vi "Panel.vi"(11 "PlatformArrayPanel in":refnum<class "PlatformArrayPanel.lvclass">) -> ()   [LabVIEW 2020, in "PicoG-App.lvlib" / "PlatformArrayPanel.lvclass"]
uses:
  PlatformArrayPanel.lvclass
  C:/Program Files (x86)/National Instruments/LabVIEW 2020/vi.lib/IlluminatedG/IG OOPanel/OOPanel/Panel/Panel.lvclass
  <vilib>/IlluminatedG/IG OOPanel/OOPanel/Panel/Basic UI State.ctl
  PlatformArrayPanel.lvclass/PlatformArrayPanel.ctl
  Builds/picoG/ppl/PicoG-Core.lvlibp/PicoG-Processor/PicoG-Core/DeployPlatform/DeployPlatform.lvclass
  <vilib>/IlluminatedG/IG OOPanel/OOPanel/Panel/Panel.lvclass
  <vilib>/IlluminatedG/IG OOPanel/OOPanel/OOPanel.lvlib
  C:/Program Files (x86)/National Instruments/LabVIEW 2020/vi.lib/IlluminatedG/IG OOPanel/OOPanel/ArrayPanel/ArrayPanel.lvclass
  C:/dev/Vireo/PicoG/PicoG-App/PlatformArrayPanel/PlatformArrayPanel.lvclass
panel:
  out "Name":string
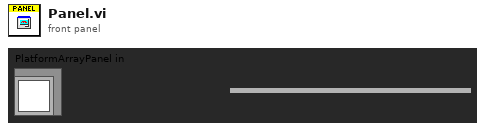
[diagram p1: front panel]
types:
  T1 = typedef "OOPanel.lvlib/Panel.lvclass/Basic UI State.ctl" = enum16{"Init", "Run", "Close"}
  T2 = typedef "PicoG-App.lvlib/PlatformArrayPanel.lvclass/Panel Events.ctl" = cluster{"Set Highlighted":refnum<user-event>}
  T3 = typedef "OOPanel.lvlib/Panel.lvclass/Panel Events.ctl" = cluster{"Visbility":refnum<user-event>, "Close":refnum<user-event>}
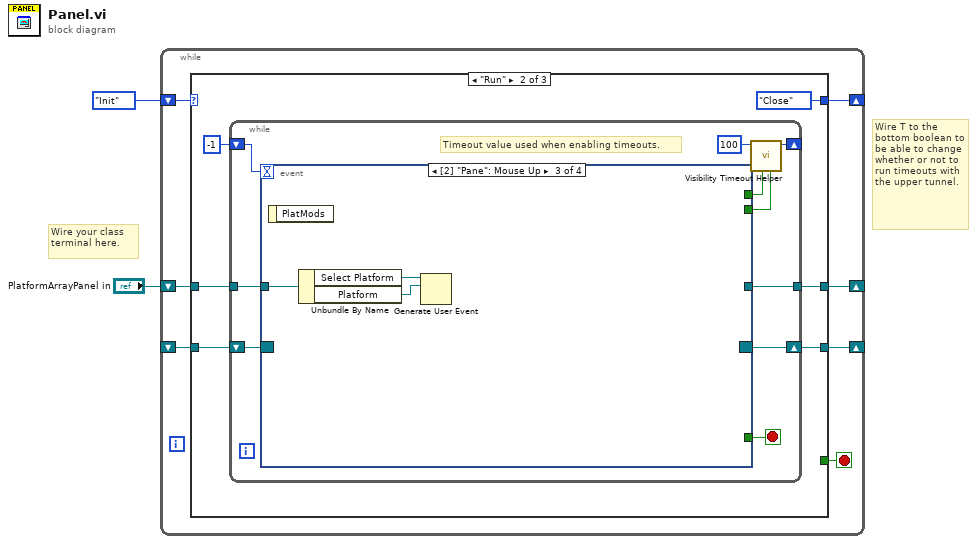
[diagram p0: block diagram]
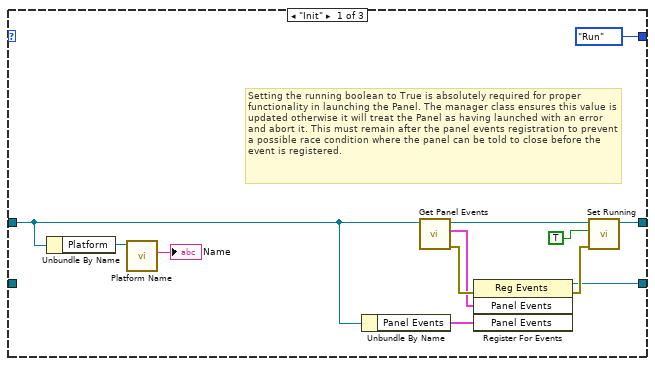
[diagram p2: hidden frame]
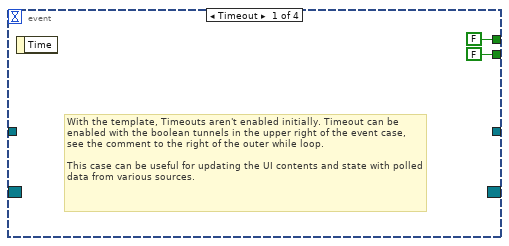
[diagram p3: hidden frame]
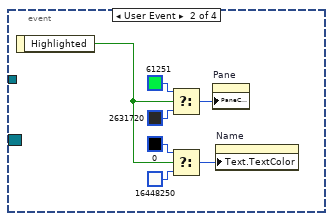
[diagram p4: hidden frame]
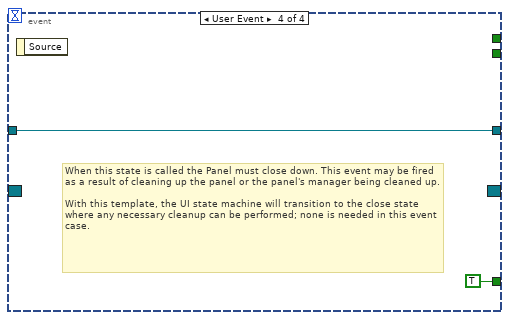
[diagram p5: hidden frame]
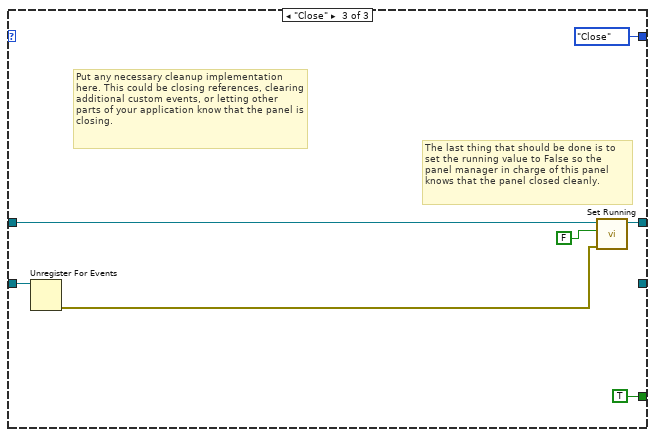
[diagram p6: hidden frame]
diagram:
  # "Wire T to the bottom boolean to be able to change whether or not to run timeouts with the upper tunnel."
  # "Wire your class terminal here."
  n1 = while {
    shift-right: [w8] -> _
    shift-left: _ -> [w9]
    shift-right: [w6] -> _
    shift-left: Basic_UI_State."Init" ("Basic UI State") -> [w7]
    shift-right: [w4] -> _
    shift-left: "PlatformArrayPanel in" -> [w3]
    stop <- w5 stop-if-true
    n2 = case shown="\"Run\"" w7 {
      tunnel: w9 -> [_ w27 w54]
      tunnel: [w15 w25 _] -> w8
      tunnel: [Basic_UI_State."Run" ("Basic UI State") Basic_UI_State."Close" ("Basic UI State") Basic_UI_State."Close" ("Basic UI State")] -> w6
      tunnel: [_ _ TRUE] -> w5
      tunnel: [w14 w22 w52] -> w4
      tunnel: w3 -> [w11 w23 w53]
      frame "Init" {
        # "Setting the running boolean to True is absolutely required for proper functionality in launching the Panel. The manager class ensures this value is updated otherwise it will treat the Panel as having launched with an error and abort it. This must remain after the panel events registration to prevent a possible race condition where the panel can be told to close before the event is registered."
        n3 = Unbundle By Name(w11) -> ("Platform"=w12:refnum<class "DeployPlatform.lvclass">)
        n4 = call-dynamic "Platform Name.vi"("DeployTarget in"=w12) -> ("Platform Name"=→"Name":string)  [unwired: 8 in, 2 out]
        n5 = Unbundle By Name(w11) -> ("Panel Events"=w10:T2)
        n6 = call <vilib>:"Get Panel Events.vi"("Panel in"=w11) -> ("error out"=w21:errorcluster, "Panel Events"=w17:T3, "Panel out"=w18:refnum<class "PlatformArrayPanel.lvclass">)  [unwired: 8 in]
        n7 = register-events(error in=w21, w17, w10) -> (reference out=w15:refnum<event-registration>, error out=w19:errorcluster)  [unwired: 1 in]
        n8 = call <vilib>:"Set Running.vi"("error in (no error)"=w19, "Running"=TRUE, "Panel in"=w18) -> ("Panel out"=w14:refnum<class "PlatformArrayPanel.lvclass">)  [unwired: 7 in, 1 out]
      }
      frame "Run" {
        n9 = while {
          shift-right: [w33] -> w25
          shift-left: w27 -> [w34]
          shift-right: [w36] -> _
          shift-left: -1 ("Timeout") -> [w35]
          tunnel: w23 -> [w29]
          tunnel: [w28] -> w22
          stop <- w30 stop-if-true
          # "Timeout value used when enabling timeouts."
          n10 = event shown="[2] \"Pane\": Mouse Up" {
            selector: w34 -> [_ _ _ _]
            dyn-events: [_ _ _ _] -> w33
            timeout: w35 -> [_ _ _ _]
            tunnel: [FALSE _ _ _] -> w32
            tunnel: [FALSE _ _ _] -> w31
            tunnel: [_ _ _ TRUE] -> w30
            tunnel: w29 -> [_ _ w49 w50]
            tunnel: [_ _ _ w50] -> w28
            event Timeout {
              # "With the template, Timeouts aren't enabled initially. Timeout can be enabled with the boolean tunnels in the upper right of the event case, see the comment to the right of the outer while loop.\n\nThis case can be useful for updating the UI contents and state with polled data from various sources."
              n11 = event-data() -> ()  [unwired: 1 in, 1 out]
            }
            event User Event {
              n12 = event-data() -> ("Highlighted"=w40:bool)  [unwired: 1 in]
              n13 = Select(t=u32 61251, s=w40, f=u32 2631720) -> (s? t:f=w44:u32)
              n14 = Select(t=u32 0, s=w40, f=u32 16448250) -> (s? t:f=w41:u32)
              n15 = property on="Pane" class="Pane"("PaneColor"=w44) -> ()  [unwired: 2 in, 2 out]
              n16 = property on="Name" class="Str"("Text.TextColor"=w41) -> ()  [unwired: 2 in, 2 out]
            }
            event Mouse Up {
              n17 = event-data() -> ()  [unwired: 1 in, 1 out]
              n18 = Unbundle By Name(w49) -> ("Select Platform"=w48:refnum<user-event>, "Platform"=w47:refnum<class "DeployPlatform.lvclass">)
              n19 = Generate User Event(user event=w48, event data cluster=w47) -> ()  [unwired: 2 in, 2 out]
            }
            event User Event {
              # "When this state is called the Panel must close down. This event may be fired as a result of cleaning up the panel or the panel's manager being cleaned up.\n\nWith this template, the UI state machine will transition to the close state where any necessary cleanup can be performed; none is needed in this event case."
              n20 = event-data() -> ()  [unwired: 1 in, 1 out]
            }
          }
          n21 = call <vilib>:"Visibility Timeout Helper.vi"("Update?"=w31, "Use Timeout?"=w32, "Visible Timeout mS"=100) -> ("Timeout"=w36:i32)  [unwired: 8 in]
        }
      }
      frame "Close" {
        # "Put any necessary cleanup implementation here. This could be closing references, clearing additional custom events, or letting other parts of your application know that the panel is closing."
        # "The last thing that should be done is to set the running value to False so the panel manager in charge of this panel knows that the panel closed cleanly."
        n22 = Unregister For Events(event registration refnum=w54) -> (error out=w56:errorcluster)  [unwired: 1 in]
        n23 = call <vilib>:"Set Running.vi"("error in (no error)"=w56, "Running"=FALSE, "Panel in"=w53) -> ("Panel out"=w52:refnum<class "PlatformArrayPanel.lvclass">)  [unwired: 7 in, 1 out]
      }
    }
  }
